vi "B value From itx.vi"(10 "B Field Name":string, 11 "file (use dialog)":path) -> (3 "Numeric":dbl)   [LabVIEW 2016]
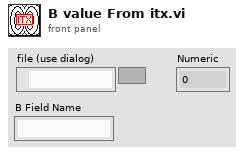
[diagram p1: front panel]
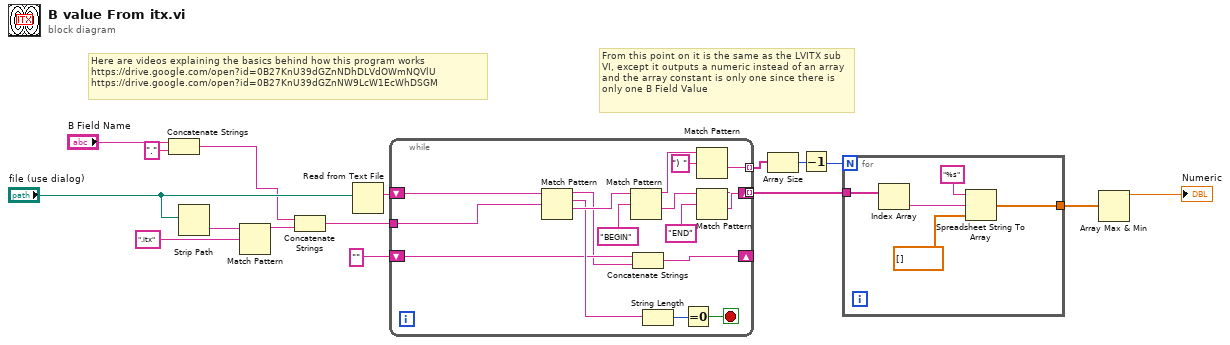
[diagram p0: block diagram]
diagram:
  # "Here are videos explaining the basics behind how this program works\nhttps://drive.google.com/open?id=0B27KnU39dGZnNDhDLVdOWmNQVlU\nhttps://drive.google.com/open?id=0B27KnU39dGZnNW9LcW1EcWhDSGM"
  # "From this point on it is the same as the LVITX sub VI, except it outputs a numeric instead of an array and the array constant is only one since there is only one B Field Value"
  n1 = Concatenate Strings("B Field Name", "." ("string")) -> (w1:string)
  n2 = Strip Path(path="file (use dialog)") -> (name=w6:string)  [unwired: 1 out]
  n3 = Match Pattern(string=w6, regular expression=".itx") -> (before substring=w5:string)  [unwired: 1 in, 3 out]
  n4 = Concatenate Strings(w1, w5) -> (w4:string)
  n5 = Read from Text File(file (use dialog)="file (use dialog)") -> (text=w14:string)  [unwired: 2 in, 4 out]
  n6 = while {
    tunnel: [w18] -> w12 mode=indexing
    shift-right: [w31] -> _
    shift-left: w14 -> [w20]
    tunnel: [w27] -> w11 mode=indexing
    shift-right: [w23] -> _
    shift-left: "" ("regular expression") -> [w22]
    tunnel: w4 -> [w17]
    stop <- w28 stop-if-true
    n7 = Match Pattern(string=w20, regular expression=w17) -> (before substring=w21:string, match substring=w30:string, after substring=w33:string)  [unwired: 2 out]
    n8 = Match Pattern(string=w33, regular expression="BEGIN" ("regular expression 2")) -> (before substring=w19:string, after substring=w32:string)  [unwired: 3 out]
    n9 = Concatenate Strings(w22, w21) -> (w23:string)
    n10 = String Length(string=w30) -> (length=w29:i32)
    n11 = Equal To 0?(x=w29) -> (x = 0?=w28:bool)
    n12 = Match Pattern(string=w19, regular expression=") ") -> (after substring=w27:string)  [unwired: 4 out]
    n13 = Match Pattern(string=w32, regular expression="END" ("regular expression 3")) -> (before substring=w18:string, after substring=w31:string)  [unwired: 3 out]
  }
  n14 = Array Size(array=w11) -> (size(s)=w10:i32)
  n15 = Decrement(x=w10) -> (x-1=w9:i32)
  n16 = for {
    N: w9 -> [_]
    tunnel: w12 -> [w38]
    tunnel: [w34] -> w15
    n17 = Index Array(array=w38) -> (element=w37:string)  [unwired: 1 in]
    n18 = Spreadsheet String To Array(format string="%s", spreadsheet string=w37, array type (2D Dbl)=dbl[] []) -> (array=w34:dbl[])  [unwired: 1 out]
  }
  n19 = Array Max & Min(array=w15) -> (max value=→"Numeric":dbl)  [unwired: 3 out]
